vi "Adb Restart App.vi"(8 "error in (no error)":errorcluster, 11 "AdbBridge in":refnum<class "AdbBridge.lvclass">) -> (0 "error out":errorcluster, 3 "AdbBridge out":refnum<class "AdbBridge.lvclass">)   [LabVIEW 2016, in "AdbBridge.lvclass"]
uses:
  AdbBridge.lvclass
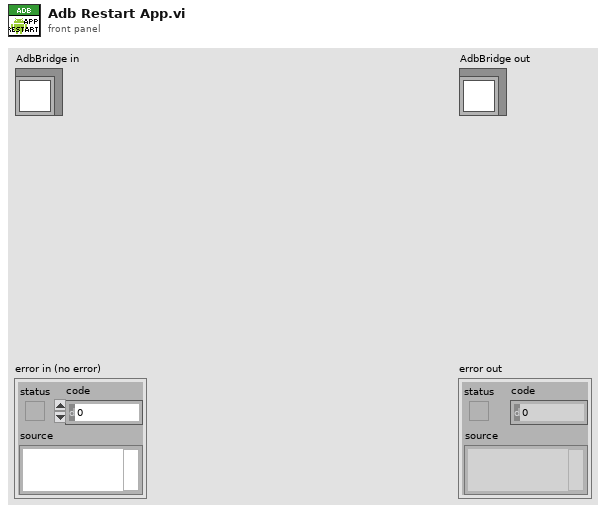
[diagram p1: front panel]
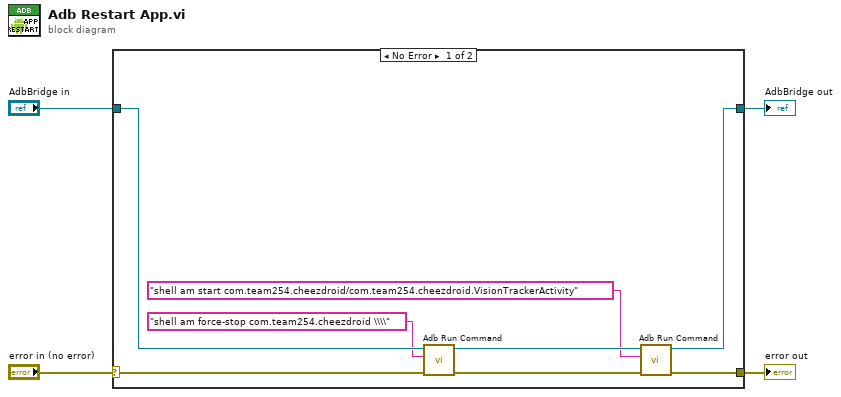
[diagram p0: block diagram]
diagram:
  n1 = case shown="No Error" "error in (no error)" {
    selector: "error in (no error)" -> [w10 w14]
    tunnel: [w8 w14] -> w3
    tunnel: [w7 w13] -> w1
    tunnel: "AdbBridge in" -> [w12 w13]
    frame No Error {
      n2 = call "Adb Run Command.vi"("error in (no error)"=w10, "args"="shell am force-stop com.team254.cheezdroid \\\\", "AdbBridge in"=w12) -> ("error out"=w9:errorcluster, "AdbBridge out"=w6:refnum<class "AdbBridge.lvclass">)  [unwired: 7 in]
      n3 = call "Adb Run Command.vi"("error in (no error)"=w9, "args"="shell am start com.team254.cheezdroid/com.team254.cheezdroid.VisionTrackerActivity", "AdbBridge in"=w6) -> ("error out"=w8:errorcluster, "AdbBridge out"=w7:refnum<class "AdbBridge.lvclass">)  [unwired: 7 in]
    }
    frame Error {
    }
  }
  "error out" <- w3
  "AdbBridge out" <- w1
